vi "TCP Read.vi"(8 "error in (no error)":errorcluster, 11 "HPS17000 Refs in":refnum<class "HPS-17000.lvclass">[](array[class])) -> (0 "error out":errorcluster, 1 "last timestamp":i64, 2 "measurement array":T1[](array[typedef]), 3 "HPS17000 Refs out":refnum<class "HPS-17000.lvclass">[](array[class]))   [LabVIEW 2023, in "HPS-17000-PowerModule.lvlib" / "HPS-17000-PowerModule.lvclass"]
uses:
  HPS-17000-PowerModule.lvclass
  <instrlib>/HPS-17000/HPS-17000.lvclass
  builds/PowerModuleInterface/PowerModuleInterface.lvlibp/Classes/PowerModule_interface/Measurements.ctl
  <instrlib>/HPS-17000/Internal/Read Measurement Multi.vi
  HPS-17000-PowerModule.lvclass/HPS-17000-PowerModule.ctl
  builds/PowerModuleInterface/PowerModuleInterface.lvlibp/Classes/PowerModule_interface/PowerModuleInterface.lvclass
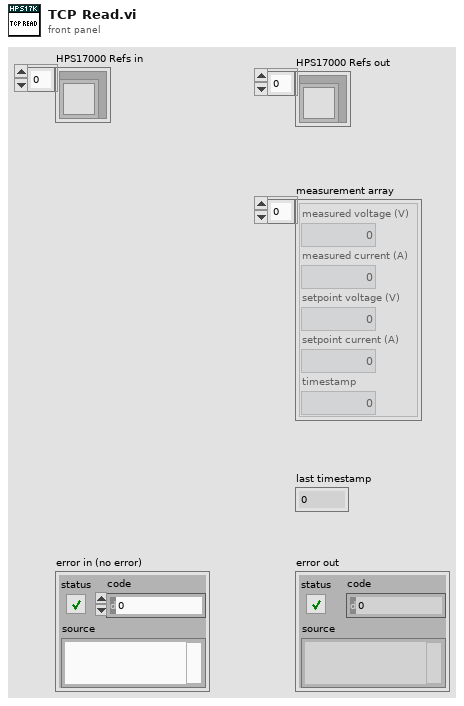
[diagram p1: front panel]
types:
  T1 = typedef "PowerModuleInterface.lvlibp/PowerModuleInterface.lvclass/Measurements.ctl" = cluster{"measured voltage (V)":dbl, "measured current (A)":dbl, "setpoint voltage (V)":dbl, "setpoint current (A)":dbl, "timestamp":dbl}
  T2 = typedef "NI_BC_client.lvlib/MStream_grpc_CyclerMeasurement.ctl" = cluster{"measured_voltage":sgl, "measured_current":sgl, "setpoint_voltage":sgl, "setpoint_current":sgl, "timestamp":i64}
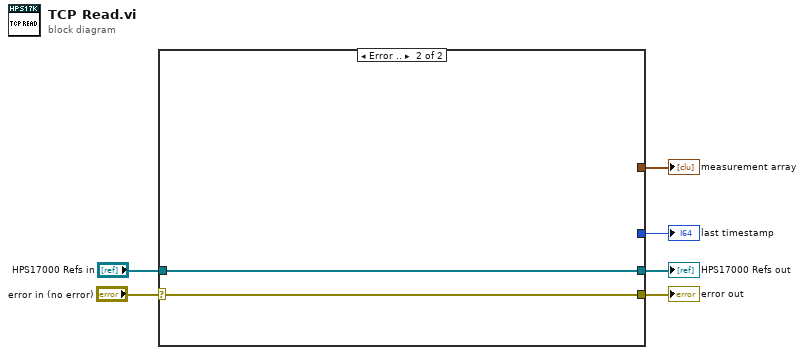
[diagram p0: block diagram]
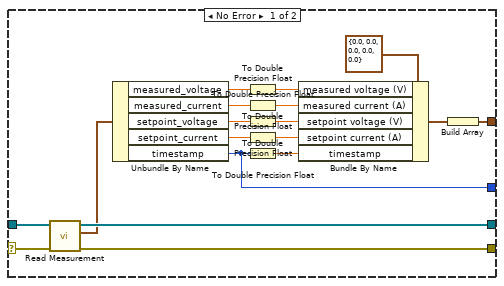
[diagram p2: hidden frame]
diagram:
  n1 = case shown="Error .." "error in (no error)" {
    selector: "error in (no error)" -> [w7 w25]
    tunnel: [w23 w26] -> w6
    tunnel: "HPS17000 Refs in" -> [w22 w26]
    tunnel: [w21 _] -> w4
    tunnel: [w9 _] -> w3
    tunnel: [w8 w25] -> w2
    frame No Error {
      n2 = call-poly <instrlib>:"Read Measurement.vi"("error in"=w7, "cycler refs in"=w22) -> ("error out"=w8:errorcluster, "aggregated cycler measurements"=w19:T2, "cycler refs out"=w23:refnum<class "HPS-17000.lvclass">[])  [unwired: 7 in]
      n3 = Unbundle By Name(w19) -> ("measured_voltage"=w12:sgl, "measured_current"=w10:sgl, "setpoint_voltage"=w11:sgl, "setpoint_current"=w13:sgl, "timestamp"=w21:i64)
      n4 = To Double Precision Float(number=w12) -> (double precision float=w14:dbl)
      n5 = To Double Precision Float(number=w10) -> (double precision float=w15:dbl)
      n6 = To Double Precision Float(number=w11) -> (double precision float=w16:dbl)
      n7 = To Double Precision Float(number=w13) -> (double precision float=w17:dbl)
      n8 = To Double Precision Float(number=w21) -> (double precision float=w24:dbl)
      n9 = Bundle By Name(cluster=T1 {"measured voltage (V)"=0.0, "measured current (A)"=0.0, "setpoint voltage (V)"=0.0, "setpoint current (A)"=0.0, "timestamp"=0.0} ("Measurements"), "measured voltage (V)"=w14, "measured current (A)"=w15, "setpoint voltage (V)"=w16, "setpoint current (A)"=w17, "timestamp"=w24) -> (w18:T1)
      n10 = Build Array(w18) -> (w9:T1[])
    }
    frame Error {
    }
  }
  "HPS17000 Refs out" <- w6
  "last timestamp" <- w4
  "measurement array" <- w3
  "error out" <- w2
